vi "MoticApi.vi"() -> ()   [LabVIEW 2012]
uses:
  MoticApi/MoticApi.lvlib
  <vilib>/picture/picture.llb/imagedata.ctl
panel:
  in  "Reset ROI":bool
  in  "Right":i32
  in  "Bottom":i32
  in  "Left":i32
  in  "Top":i32
  out "Max height":i32=486
  out "Max width":i32=648
  out "Bits per component":i32
  out "Components per pixel":i32
  in  "Activate cooler":bool
  out "Cooler available?":bool
  out "Camera connected":bool
  out "Frame format":u32(ring) items=["GRBG", "BGGR", "GBRG", "RGGB", "RGB", "BGR", "Monochrome"]
  out "Camera type":u32(ring) items=["Unknown", "MC1001", "MC2001", "MC3001", "MC2001B", "MC1002", "MC2002", "MA205", "MA285", "MA252", "Swift MC1002", "MD3300: deprecated Since MA252 added", "MC5001", "MC3111", "MC3222", "MC3022", "Swift MC3001", "Swift MC3222", "Swift MC3111", "MA282", "MC352+: Not available at present", "MC3521: Not available at present", "MC10M"]
  in  "Trigger type":u32(ring) items=["Free", "Software", "Hardware-Rise", "Hardware-Fall"]
  out "Temperature data available?":bool
  out "Relative Humidity":dbl
  out "Ambient Temperature":dbl
  out "Sensor temperature":dbl
  in  "Resolution":i32(ring) items=["2592 x 1944", "1296 x 972", "648 x 486"]
  in  "Frequency index":i32(slide)=3 min=0 max=8 step=1 scale=0.0..8.0
  in  "Exposure, ms":sgl(slide)=0.14 min=0.14 max=5674.29 step=1 scale=0.14000000059604645..5674.2919921875
  out "Current height":i32=486
  out "Current width":i32=648
  in  "Acquisition enabled":bool
  in  "Blue Gain":sgl(slide)=1.0 min=1 max=128 step=0.125 scale=1.0..128.0
  in  "Green Gain":sgl(slide)=1.0 min=1 max=128 step=0.125 scale=1.0..128.0
  in  "Red Gain":sgl(slide)=1.0 min=1 max=128 step=0.125 scale=1.0..128.0
  in  "Blue Offset":i32(slide) min=-255 max=255 step=1 scale=-255.0..255.0
  in  "Green Offset":i32(slide) min=-255 max=255 step=1 scale=-255.0..255.0
  in  "Red Offset":i32(slide) min=-255 max=255 step=1 scale=-255.0..255.0
  out "Image":T1(plugin-control)
  in  "stop":bool
  out "2D Picture":picture
  out "height array out":i32[](array[numeric])=[1944, 972, 486]
  out "width array out":i32[](array[numeric])=[2592, 1296, 648]
  out "error out":errorcluster
  # "ROI configuration"
  # "0 - fastest"
  # "Color Gain"
  # "Color Offset"
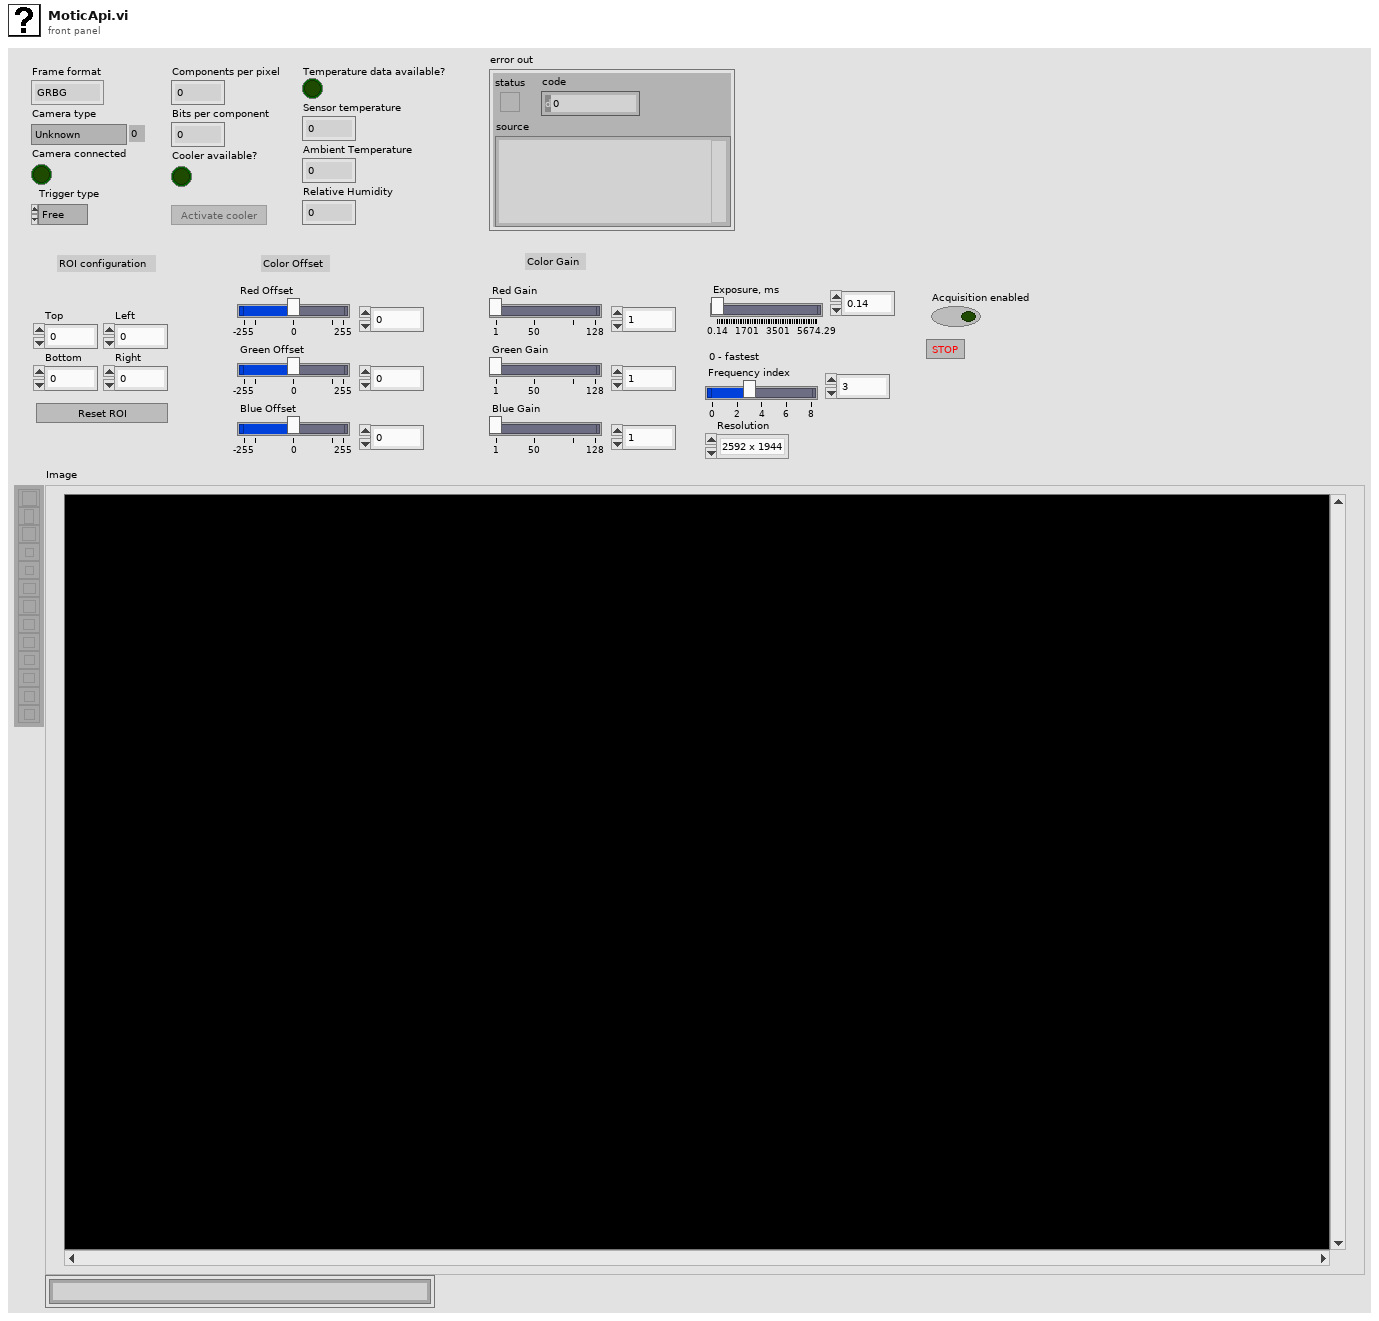
[diagram p1: front panel]
types:
  T1 = typedef "IMAQ Image.ctl" = refnum<image>
  T2 = enum8{"Enabled", "Disabled", "Disabled and Grayed Out"}
  T3 = typedef "Image Type" = u32
  T4 = cluster{"left":i16, "top":i16, "right":i16, "bottom":i16}
  T5 = typedef "imagedata.ctl" = cluster{"image type":i32, "image depth":i32, "image":u8[], "mask":u8[], "colors":u32[], "Rectangle":cluster{"left":i16, "top":i16, "right":i16, "bottom":i16}}
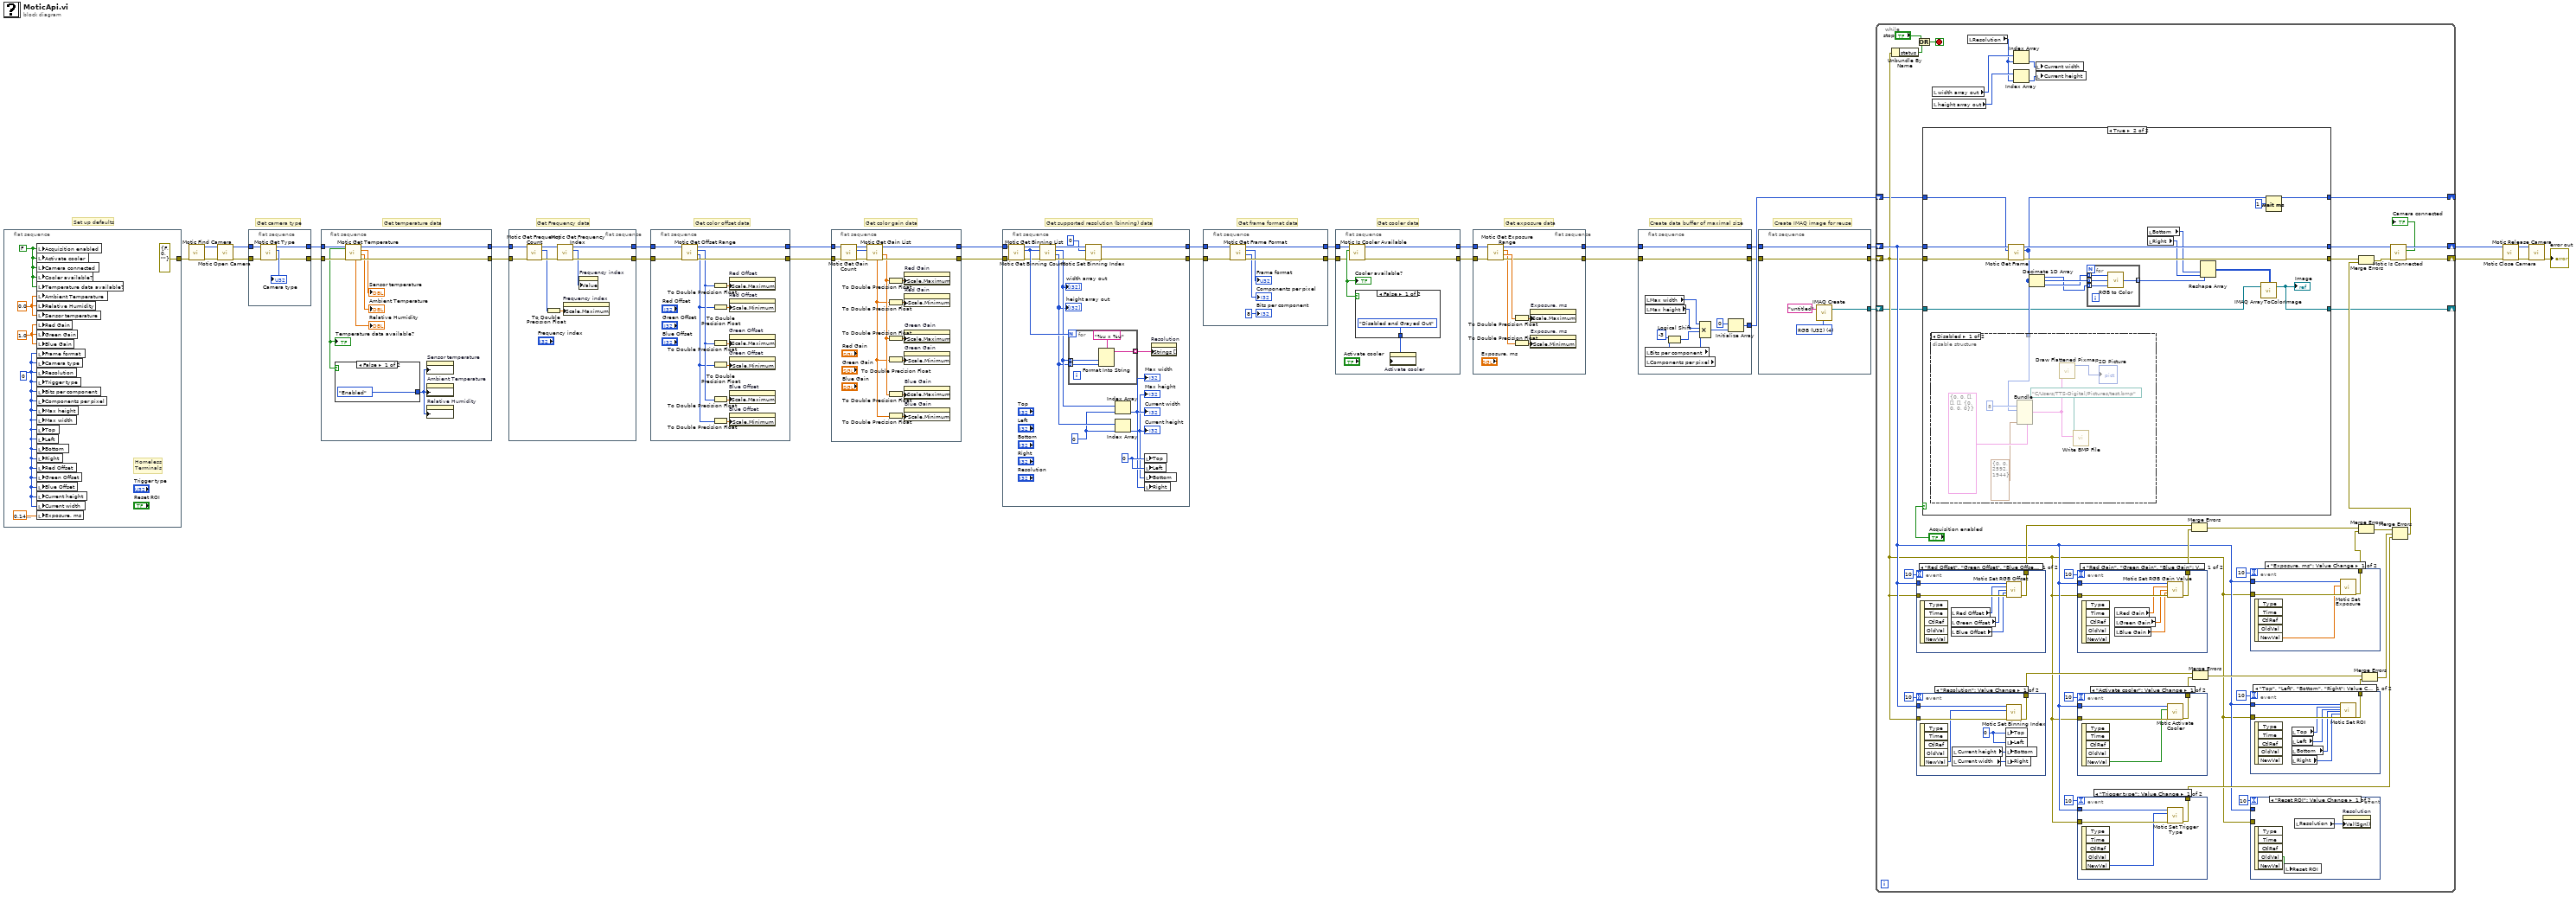
[diagram p0: block diagram]
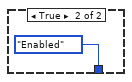
[diagram p2: hidden frame]
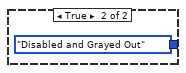
[diagram p3: hidden frame]
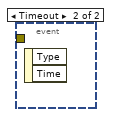
[diagram p4: hidden frame]
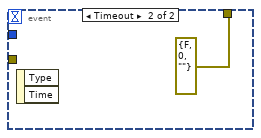
[diagram p5: hidden frame]
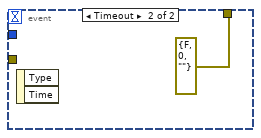
[diagram p6: hidden frame]
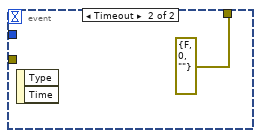
[diagram p7: hidden frame]
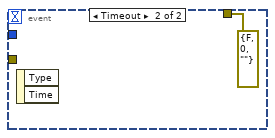
[diagram p8: hidden frame]
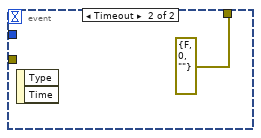
[diagram p9: hidden frame]
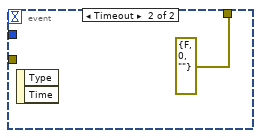
[diagram p10: hidden frame]
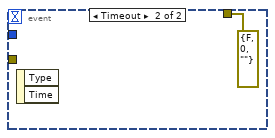
[diagram p13: hidden frame]
diagram:
  # "Set up defaults"
  # "Create IMAQ image for reuse"
  # "Create data buffer of maximal size"
  # "Get camera type"
  # "Get exposure data"
  # "Get cooler data"
  # "Get frame format data"
  # "Get supported resolution (binning) data"
  # "Get color gain data"
  # "Get color offset data"
  # "Get Frequency data"
  # "Get temperature data"
  n1 = flat-sequence {
    tunnel: [errorcluster {"status"=FALSE, "code"=0, "source"=""} ("error in (no error)")] -> w7
    frame #0 {
      w35 = sgl 1.0 ("Red Gain")
      w36 = 0
      w39 = 0.0 ("Ambient Temperature")
      w37 = FALSE ("Acquisition enabled")
      # "Homeless\nTerminals"
      n2 = local write "Acquisition enabled"(w37) -> ()
      n3 = local write "Activate cooler"(w37) -> ()
      n4 = local write "Camera connected"(w37) -> ()
      n5 = local write "Cooler available?"(w37) -> ()
      n6 = local write "Temperature data available?"(w37) -> ()
      n7 = local write "Ambient Temperature"(w39) -> ()
      n8 = local write "Relative Humidity"(w39) -> ()
      n9 = local write "Sensor temperature"(w39) -> ()
      n10 = local write "Red Gain"(w35) -> ()
      n11 = local write "Green Gain"(w35) -> ()
      n12 = local write "Blue Gain"(w35) -> ()
      n13 = local write "Frame format"(w36) -> ()
      n14 = local write "Camera type"(w36) -> ()
      n15 = local write "Resolution"(w36) -> ()
      n16 = local write "Trigger type"(w36) -> ()
      n17 = local write "Bits per component"(w36) -> ()
      n18 = local write "Components per pixel"(w36) -> ()
      n19 = local write "Max height"(w36) -> ()
      n20 = local write "Max width"(w36) -> ()
      n21 = local write "Top"(w36) -> ()
      n22 = local write "Left"(w36) -> ()
      n23 = local write "Bottom"(w36) -> ()
      n24 = local write "Right"(w36) -> ()
      n25 = local write "Red Offset"(w36) -> ()
      n26 = local write "Green Offset"(w36) -> ()
      n27 = local write "Blue Offset"(w36) -> ()
      n28 = local write "Current height"(w36) -> ()
      n29 = local write "Current width"(w36) -> ()
      n30 = local write "Exposure, ms"(sgl 0.14 ("Exposure, ms")) -> ()
    }
  }
  n31 = call "Motic Find Camera.vi"("error in (no error)"=w7) -> ("error out"=w14:errorcluster, "camera out"=w17:i32)  [unwired: 9 in]
  n32 = call "Motic Open Camera.vi"("error in (no error)"=w14, "camera"=w17) -> ("error out"=w15:errorcluster, "camera out"=w16:i32)  [unwired: 8 in]
  n33 = flat-sequence {
    tunnel: [w44] -> w19
    tunnel: [w43] -> w18
    tunnel: w16 -> [w42]
    tunnel: w15 -> [w41]
    frame #0 {
      n34 = call "Motic Get Type.vi"("error in (no error)"=w41, "camera"=w42) -> ("error out"=w43:errorcluster, "camera type"=→"Camera type":u32, "camera out"=w44:i32)  [unwired: 7 in]
    }
  }
  n35 = flat-sequence {
    tunnel: w19 -> [w54]
    tunnel: w18 -> [w53]
    tunnel: [w52] -> w25
    tunnel: [w51] -> w24
    frame #0 {
      n36 = call "Motic Get Temperature.vi"("error in (no error)"=w53, "camera"=w54) -> ("error out"=w51:errorcluster, "ambient temperature out"=→"Ambient Temperature":sgl, "sensor surface temperature out"=→"Sensor temperature":sgl, "camera out"=w52:i32, "relative humidity out"=→"Relative Humidity":sgl, "is temperature data available?"=w47:bool)  [unwired: 4 in]
      "Temperature data available?" <- w47
      n37 = case shown="False" w47 {
        tunnel: [T2."Enabled" ("Disabled") T2."Disabled and Grayed Out" ("Disabled")] -> w46
        frame False {
        }
        frame True {
        }
      }
      n38 = property on="Sensor temperature" class="DigNum (strict)"("DisabledEnum"=w46) -> ()  [unwired: 2 in, 2 out]
      n39 = property on="Ambient Temperature" class="DigNum (strict)"("DisabledEnum"=w46) -> ()  [unwired: 2 in, 2 out]
      n40 = property on="Relative Humidity" class="DigNum (strict)"("DisabledEnum"=w46) -> ()  [unwired: 2 in, 2 out]
    }
  }
  n41 = flat-sequence {
    tunnel: [w63] -> w27
    tunnel: [w62] -> w26
    tunnel: w25 -> [w58]
    tunnel: w24 -> [w57]
    frame #0 {
      n42 = call "Motic Get Frequency Count.vi"("error in (no error)"=w57, "camera"=w58) -> ("error out"=w64:errorcluster, "frequency count"=w60:i32, "camera out"=w65:i32)  [unwired: 7 in]
      n43 = To Double Precision Float(number=w60) -> (double precision float=w61:dbl)
      n44 = call "Motic Get Frequency Index.vi"("error in (no error)"=w64, "camera"=w65) -> ("error out"=w62:errorcluster, "frequency index"=w59:i32, "camera out"=w63:i32)  [unwired: 7 in]
      n45 = property on="Frequency index" class="Slide (strict)"("Scale.Maximum"=w61) -> ()  [unwired: 2 in, 2 out]
      n46 = property on="Frequency index" class="Slide (strict)"("Value"=w59) -> ()  [unwired: 2 in, 2 out]
    }
  }
  n47 = flat-sequence {
    tunnel: [w77] -> w2
    tunnel: [w76] -> w1
    tunnel: w27 -> [w67]
    tunnel: w26 -> [w66]
    frame #0 {
      n48 = call "Motic Get Offset Range.vi"("error in (no error)"=w66, "camera"=w67) -> ("error out"=w76:errorcluster, "min out"=w68:i32, "max out"=w69:i32, "camera out"=w77:i32)  [unwired: 6 in]
      n49 = To Double Precision Float(number=w69) -> (double precision float=w74:dbl)
      n50 = To Double Precision Float(number=w68) -> (double precision float=w75:dbl)
      n51 = To Double Precision Float(number=w69) -> (double precision float=w72:dbl)
      n52 = To Double Precision Float(number=w68) -> (double precision float=w73:dbl)
      n53 = To Double Precision Float(number=w69) -> (double precision float=w70:dbl)
      n54 = To Double Precision Float(number=w68) -> (double precision float=w71:dbl)
      n55 = property on="Red Offset" class="Slide (strict)"("Scale.Maximum"=w74) -> ()  [unwired: 2 in, 2 out]
      n56 = property on="Red Offset" class="Slide (strict)"("Scale.Minimum"=w75) -> ()  [unwired: 2 in, 2 out]
      n57 = property on="Green Offset" class="Slide (strict)"("Scale.Maximum"=w72) -> ()  [unwired: 2 in, 2 out]
      n58 = property on="Green Offset" class="Slide (strict)"("Scale.Minimum"=w73) -> ()  [unwired: 2 in, 2 out]
      n59 = property on="Blue Offset" class="Slide (strict)"("Scale.Maximum"=w70) -> ()  [unwired: 2 in, 2 out]
      n60 = property on="Blue Offset" class="Slide (strict)"("Scale.Minimum"=w71) -> ()  [unwired: 2 in, 2 out]
    }
  }
  n61 = flat-sequence {
    tunnel: w2 -> [w92]
    tunnel: w1 -> [w91]
    tunnel: [w81] -> w3
    tunnel: [w80] -> w4
    frame #0 {
      n62 = call "Motic Get Gain Count.vi"("error in (no error)"=w91, "camera"=w92) -> ("error out"=w88:errorcluster, "gain count"=w90:i32, "camera out"=w89:i32)  [unwired: 7 in]
      n63 = call "Motic Get Gain List.vi"("error in (no error)"=w88, "gain count"=w90, "camera"=w89) -> ("error out"=w81:errorcluster, "max gain"=w79:sgl, "camera out"=w80:i32, "min gain"=w78:sgl)  [unwired: 4 in, 1 out]
      n64 = To Double Precision Float(number=w79) -> (double precision float=w86:dbl)
      n65 = To Double Precision Float(number=w78) -> (double precision float=w87:dbl)
      n66 = To Double Precision Float(number=w79) -> (double precision float=w84:dbl)
      n67 = To Double Precision Float(number=w78) -> (double precision float=w85:dbl)
      n68 = To Double Precision Float(number=w79) -> (double precision float=w82:dbl)
      n69 = To Double Precision Float(number=w78) -> (double precision float=w83:dbl)
      n70 = property on="Red Gain" class="Slide (strict)"("Scale.Maximum"=w86) -> ()  [unwired: 2 in, 2 out]
      n71 = property on="Red Gain" class="Slide (strict)"("Scale.Minimum"=w87) -> ()  [unwired: 2 in, 2 out]
      n72 = property on="Green Gain" class="Slide (strict)"("Scale.Maximum"=w84) -> ()  [unwired: 2 in, 2 out]
      n73 = property on="Green Gain" class="Slide (strict)"("Scale.Minimum"=w85) -> ()  [unwired: 2 in, 2 out]
      n74 = property on="Blue Gain" class="Slide (strict)"("Scale.Maximum"=w82) -> ()  [unwired: 2 in, 2 out]
      n75 = property on="Blue Gain" class="Slide (strict)"("Scale.Minimum"=w83) -> ()  [unwired: 2 in, 2 out]
    }
  }
  n76 = flat-sequence {
    tunnel: [w105] -> w23
    tunnel: [w104] -> w22
    tunnel: w4 -> [w101]
    tunnel: w3 -> [w100]
    frame #0 {
      w95 = 0 ("index")
      w96 = 0 ("Top")
      n77 = call "Motic Get Binning Count.vi"("error in (no error)"=w100, "camera"=w101) -> ("error out"=w102:errorcluster, "binning count"=w106:i32, "camera out"=w103:i32)  [unwired: 7 in]
      n78 = call "Motic Get Binning List.vi"("error in (no error)"=w102, "binning count"=w106, "camera"=w103) -> ("error out"=w108:errorcluster, "height array out"=w97:i32[], "width array out"=w98:i32[], "camera out"=w109:i32)  [unwired: 5 in]
      "width array out" <- w98
      "height array out" <- w97
      n79 = for {
        N: w106 -> [_]
        tunnel: w98 -> [w112] mode=indexing
        tunnel: w97 -> [w111] mode=indexing
        tunnel: [w110] -> w99 mode=indexing
        n80 = Format Into String(format string="%u x %u", w112, w111) -> (resulting string=w110:string)  [unwired: 2 in, 1 out]
      }
      n81 = call "Motic Set Binning Index.vi"("error in (no error)"=w108, "idx"=0, "camera"=w109) -> ("error out"=w104:errorcluster, "camera out"=w105:i32)  [unwired: 7 in]
      n82 = Index Array(array=w98, index=w95) -> (element=w94:i32)
      "Current width" <- w94
      "Max width" <- w94
      n83 = Index Array(array=w97, index=w95) -> (element=w93:i32)
      "Current height" <- w93
      "Max height" <- w93
      n84 = local write "Top"(w96) -> ()
      n85 = local write "Left"(w96) -> ()
      n86 = local write "Bottom"(w93) -> ()
      n87 = local write "Right"(w94) -> ()
      n88 = property on="Resolution" class="Ring (strict)"("Strings []"=w99) -> ()  [unwired: 2 in, 2 out]
    }
  }
  n89 = flat-sequence {
    tunnel: w23 -> [w120]
    tunnel: w22 -> [w119]
    tunnel: [w118] -> w21
    tunnel: [w117] -> w20
    frame #0 {
      n90 = call "Motic Get Frame Format.vi"("error in (no error)"=w119, "camera"=w120) -> ("error out"=w117:errorcluster, "components per pixel"=→"Components per pixel":i32, "frame format"=→"Frame format":u32, "camera out"=w118:i32)  [unwired: 6 in]
      "Bits per component" <- 8 ("bits per component")
    }
  }
  n91 = flat-sequence {
    tunnel: [w126] -> w29
    tunnel: [w125] -> w28
    tunnel: w21 -> [w123]
    tunnel: w20 -> [w122]
    frame #0 {
      n92 = call "Motic Is Cooler Available.vi"("error in (no error)"=w122, "camera"=w123) -> ("error out"=w125:errorcluster, "cooler available?"=w124:bool, "camera out"=w126:i32)  [unwired: 7 in]
      "Cooler available?" <- w124
      n93 = case shown="False" w124 {
        tunnel: [T2."Disabled and Grayed Out" ("Disabled") T2."Enabled" ("Disabled")] -> w121
        frame False {
        }
        frame True {
        }
      }
      n94 = property on="Activate cooler" class="Bool (strict)"("DisabledEnum"=w121) -> ()  [unwired: 2 in, 2 out]
    }
  }
  n95 = flat-sequence {
    tunnel: [w133] -> w6
    tunnel: [w132] -> w5
    tunnel: w29 -> [w130]
    tunnel: w28 -> [w129]
    frame #0 {
      n96 = call "Motic Get Exposure Range.vi"("error in (no error)"=w129, "camera"=w130) -> ("error out"=w132:errorcluster, "range max"=w134:sgl, "range min"=w131:sgl, "camera out"=w133:i32)  [unwired: 6 in]
      n97 = To Double Precision Float(number=w134) -> (double precision float=w135:dbl)
      n98 = To Double Precision Float(number=w131) -> (double precision float=w136:dbl)
      n99 = property on="Exposure, ms" class="Slide (strict)"("Scale.Maximum"=w135) -> ()  [unwired: 2 in, 2 out]
      n100 = property on="Exposure, ms" class="Slide (strict)"("Scale.Minimum"=w136) -> ()  [unwired: 2 in, 2 out]
    }
  }
  n101 = flat-sequence {
    tunnel: [w147] -> w12
    tunnel: [w146] -> w11
    tunnel: w6 -> [w147]
    tunnel: w5 -> [w146]
    tunnel: [w137] -> w13
    frame #0 {
      n102 = local read "Max width"() -> (w141:i32)
      n103 = local read "Max height"() -> (w138:i32)
      n104 = local read "Bits per component"() -> (w139:i32)
      n105 = local read "Components per pixel"() -> (w140:i32)
      n106 = Logical Shift(y=-3, x=w139) -> (x << y=w143:i32)
      n107 = Compound Arithmetic op=MULTIPLY(w141, w138, w143, w140) -> (w144:i32)
      n108 = Initialize Array(u8 0 ("element"), w144) -> (w137:u8[])
    }
  }
  n109 = flat-sequence {
    tunnel: [w152] -> w10
    tunnel: [w151] -> w9
    tunnel: w12 -> [w152]
    tunnel: w11 -> [w151]
    tunnel: [w148] -> w8
    frame #0 {
      w150 = T3 4 items=["Grayscale (U8)", "Grayscale (I16)", "Grayscale (SGL)", "Complex (CSG)", "RGB (U32)", "HSL (U32)", "RGB (U64)", "Grayscale (U16)"] ("Image Type")
      n110 = call "IMAQ Create"("Image Name"="untitled", "Image Type"=w150) -> ("New Image"=w148:T1)  [unwired: 3 in, 1 out]
    }
  }
  n111 = while {
    shift-right: [w178] -> w31
    shift-left: w10 -> [w167]
    shift-right: [w180] -> w30
    shift-left: w9 -> [w160]
    shift-right: [w155] -> _
    shift-left: w13 -> [w156]
    shift-right: [w153] -> _
    shift-left: w8 -> [w154]
    stop <- w157 stop-if-true
    n112 = Unbundle By Name(w160) -> ("status"=w159:bool)
    n113 = Or(x="stop", y=w159) -> (x .or. y?=w157:bool)
    n114 = event shown="[0] \"Red Offset\", \"Green Offset\", \"Blue Offset\": Value Change" {
      selector: _ -> [_ _]
      dyn-events: _ -> [_ _]
      timeout: 10 -> [_ _]
      tunnel: w167 -> [w270 _]
      tunnel: w160 -> [w269 _]
      tunnel: [w268 errorcluster {"status"=FALSE, "code"=0, "source"=""} ("error out")] -> w188
      event "Red Offset", "Green Offset", "Blue Offset": Value Change {
        n115 = event-data() -> ()  [unwired: 1 in, 5 out]
        n116 = local read "Red Offset"() -> (w267:i32)
        n117 = local read "Green Offset"() -> (w266:i32)
        n118 = local read "Blue Offset"() -> (w265:i32)
        n119 = call "Motic Set RGB Offset.vi"("camera"=w270, "r"=w267, "g"=w266, "b"=w265, "error in (no error)"=w269) -> ("error out"=w268:errorcluster)  [unwired: 9 in, 1 out]
      }
      event Timeout {
        n120 = event-data() -> ()  [unwired: 1 in, 2 out]
      }
    }
    n121 = event shown="[0] \"Resolution\": Value Change" {
      selector: _ -> [_ _]
      dyn-events: _ -> [_ _]
      timeout: 10 -> [_ _]
      tunnel: w167 -> [w220 _]
      tunnel: w160 -> [w219 _]
      tunnel: [w218 errorcluster {"status"=FALSE, "code"=0, "source"=""} ("error out")] -> w175
      event "Resolution": Value Change {
        w216 = 0 ("Top")
        n122 = event-data() -> ("NewVal"=w217:i32)  [unwired: 1 in, 4 out]
        n123 = local read "Current height"() -> (w215:i32)
        n124 = local read "Current width"() -> (w214:i32)
        n125 = local write "Top"(w216) -> ()
        n126 = local write "Left"(w216) -> ()
        n127 = local write "Bottom"(w215) -> ()
        n128 = local write "Right"(w214) -> ()
        n129 = call "Motic Set Binning Index.vi"("error in (no error)"=w219, "idx"=w217, "camera"=w220) -> ("error out"=w218:errorcluster)  [unwired: 7 in, 1 out]
      }
      event Timeout {
        n130 = event-data() -> ()  [unwired: 1 in, 2 out]
      }
    }
    n131 = case shown="True" "Acquisition enabled" {
      tunnel: [w237 w253] -> w179
      tunnel: [w236 w252] -> w191
      tunnel: w167 -> [w237 w251]
      tunnel: w160 -> [w236 w250]
      tunnel: w156 -> [w235 w241]
      tunnel: [w235 w240] -> w155
      tunnel: w154 -> [w234 w239]
      tunnel: [w234 w238] -> w153
      frame False {
      }
      frame True {
        n132 = call "Motic Get Frame.vi"("error in (no error)"=w250, "image buffer in"=w241, "camera"=w251) -> ("error out"=w252:errorcluster, "image buffer out"=w240:u8[], "camera out"=w253:i32)  [unwired: 5 in, 1 out]
        n133 = disable-structure shown="Disabled" {
          disable-tunnel: w240 -> [w254 _]
          frame Disabled {
            n134 = Bundle(cluster=T5 {"image type"=0, "image depth"=0, "image"=[], "mask"=[], "colors"=[], "Rectangle"={"left"=0, "top"=0, "right"=0, "bottom"=0}} ("image data"), "image depth"=8, "image"=w254, "Rectangle"=T4 {"left"=0, "top"=0, "right"=2592, "bottom"=1944}) -> (w258:T5)  [unwired: 3 in]
            n135 = call <vilib>:"Draw Flattened Pixmap.vi"("image data"=w258) -> ("new picture"=→"2D Picture":picture)  [unwired: 8 in]
            n136 = call <vilib>:"Write BMP File.vi"("image data"=w258, "path to BMP file"=path "C:/Users/TTS-Digital/Pictures/test.bmp") -> ()  [unwired: 8 in, 2 out]
          }
          frame Enabled {
          }
        }
        n137 = Decimate 1D Array(w240) -> (w247:u8[], w249:u8[], w248:u8[])
        n138 = for {
          tunnel: w249 -> [w263] mode=indexing
          tunnel: w247 -> [w264] mode=indexing
          tunnel: w248 -> [w262] mode=indexing
          tunnel: [w261] -> w246 mode=indexing
          n139 = call <vilib>:"RGB to Color.vi"("B"=w264, "G"=w263, "R"=w262) -> ("Color"=w261:u32)
        }
        n140 = local read "Bottom"() -> (w243:i32)
        n141 = local read "Right"() -> (w242:i32)
        n142 = Reshape Array(w246, w243, w242) -> (w245:u32[][])
        n143 = call "IMAQ ArrayToColorImage"("Image Pixels (U32)"=w245, "Image"=w239) -> ("Image Out"=w238:T1)  [unwired: 3 in, 1 out]
        "Image" <- w238
        n144 = Wait (ms)(milliseconds to wait=u32 1) -> ()  [unwired: 1 out]
      }
    }
    n145 = local read "width array out"() -> (w165:i32[])
    n146 = local read "height array out"() -> (w164:i32[])
    n147 = local read "Resolution"() -> (w163:i32)
    n148 = Index Array(array=w165, index=w163) -> (element=w162:i32)
    n149 = Index Array(array=w164, index=w163) -> (element=w161:i32)
    n150 = local write "Current width"(w162) -> ()
    n151 = local write "Current height"(w161) -> ()
    n152 = event shown="[0] \"Red Gain\", \"Green Gain\", \"Blue Gain\": Value Change" {
      selector: _ -> [_ _]
      dyn-events: _ -> [_ _]
      timeout: 10 -> [_ _]
      tunnel: w167 -> [w232 _]
      tunnel: w160 -> [w231 _]
      tunnel: [w230 errorcluster {"status"=FALSE, "code"=0, "source"=""} ("error out")] -> w189
      event "Red Gain", "Green Gain", "Blue Gain": Value Change {
        n153 = event-data() -> ()  [unwired: 1 in, 5 out]
        n154 = local read "Red Gain"() -> (w229:sgl)
        n155 = local read "Green Gain"() -> (w228:sgl)
        n156 = local read "Blue Gain"() -> (w227:sgl)
        n157 = call "Motic Set RGB Gain Value.vi"("camera"=w232, "r"=w229, "g"=w228, "b"=w227, "error in (no error)"=w231) -> ("error out"=w230:errorcluster)  [unwired: 6 in, 4 out]
      }
      event Timeout {
        n158 = event-data() -> ()  [unwired: 1 in, 2 out]
      }
    }
    n159 = event shown="[0] \"Activate cooler\": Value Change" {
      selector: _ -> [_ _]
      dyn-events: _ -> [_ _]
      timeout: 10 -> [_ _]
      tunnel: w167 -> [w212 _]
      tunnel: w160 -> [w211 _]
      tunnel: [w210 errorcluster {"status"=FALSE, "code"=0, "source"=""} ("error out")] -> w176
      event "Activate cooler": Value Change {
        n160 = event-data() -> ("NewVal"=w209:bool)  [unwired: 1 in, 4 out]
        n161 = call "Motic Activate Cooler.vi"("error in (no error)"=w211, "activate"=w209, "camera"=w212) -> ("error out"=w210:errorcluster)  [unwired: 6 in, 2 out]
      }
      event Timeout {
        n162 = event-data() -> ()  [unwired: 1 in, 2 out]
      }
    }
    n163 = event shown="[0] \"Trigger type\": Value Change" {
      selector: _ -> [_ _]
      dyn-events: _ -> [_ _]
      timeout: 10 -> [_ _]
      tunnel: w167 -> [w199 _]
      tunnel: w160 -> [w198 _]
      tunnel: [w197 errorcluster {"status"=FALSE, "code"=0, "source"=""} ("error out")] -> w168
      event "Trigger type": Value Change {
        n164 = event-data() -> ("NewVal"=w196:u32)  [unwired: 1 in, 4 out]
        n165 = call "Motic Set Trigger Type.vi"("error in (no error)"=w198, "trigger type"=w196, "camera"=w199) -> ("error out"=w197:errorcluster)  [unwired: 7 in, 1 out]
      }
      event Timeout {
        n166 = event-data() -> ()  [unwired: 1 in, 2 out]
      }
    }
    n167 = Merge Errors(w188, w189) -> (w186:errorcluster)
    n168 = Merge Errors(w175, w176) -> (w174:errorcluster)
    n169 = event shown="[0] \"Exposure, ms\": Value Change" {
      selector: _ -> [_ _]
      dyn-events: _ -> [_ _]
      timeout: 10 -> [_ _]
      tunnel: w167 -> [w225 _]
      tunnel: w160 -> [w224 _]
      tunnel: [w223 errorcluster {"status"=FALSE, "code"=0, "source"=""} ("error out")] -> w185
      event "Exposure, ms": Value Change {
        n170 = event-data() -> ("NewVal"=w222:sgl)  [unwired: 1 in, 4 out]
        n171 = call "Motic Set Exposure.vi"("error in (no error)"=w224, "exposure"=w222, "camera"=w225) -> ("error out"=w223:errorcluster)  [unwired: 7 in, 1 out]
      }
      event Timeout {
        n172 = event-data() -> ()  [unwired: 1 in, 2 out]
      }
    }
    n173 = event shown="[0] \"Top\", \"Left\", \"Bottom\", \"Right\": Value Change" {
      selector: _ -> [_ _]
      dyn-events: _ -> [_ _]
      timeout: 10 -> [_ _]
      tunnel: w167 -> [w207 _]
      tunnel: w160 -> [w206 _]
      tunnel: [w205 errorcluster {"status"=FALSE, "code"=0, "source"=""} ("error out")] -> w173
      event "Top", "Left", "Bottom", "Right": Value Change {
        n174 = event-data() -> ()  [unwired: 1 in, 5 out]
        n175 = local read "Top"() -> (w204:i32)
        n176 = local read "Left"() -> (w203:i32)
        n177 = local read "Bottom"() -> (w202:i32)
        n178 = local read "Right"() -> (w201:i32)
        n179 = call "Motic Set ROI.vi"("camera"=w207, "top"=w204, "left"=w203, "bottom"=w202, "right"=w201, "error in (no error)"=w206) -> ("error out"=w205:errorcluster)  [unwired: 8 in, 5 out]
      }
      event Timeout {
        n180 = event-data() -> ()  [unwired: 1 in, 2 out]
      }
    }
    n181 = event shown="[0] \"Reset ROI\": Value Change" {
      selector: _ -> [_ _]
      dyn-events: _ -> [_ _]
      timeout: 10 -> [_ _]
      tunnel: w167 -> [_ _]
      tunnel: w160 -> [_ _]
      event "Reset ROI": Value Change {
        n182 = event-data() -> ("OldVal"=w195:bool)  [unwired: 1 in, 4 out]
        n183 = local write "Reset ROI"(w195) -> ()
        n184 = local read "Resolution"() -> (w194:i32)
        n185 = property on="Resolution" class="Ring (strict)"("Val(Sgnl)"=w194) -> ()  [unwired: 2 in, 2 out]
      }
      event Timeout {
        n186 = event-data() -> ()  [unwired: 1 in, 2 out]
      }
    }
    n187 = Merge Errors(w186, w185) -> (w171:errorcluster)
    n188 = Merge Errors(w174, w173) -> (w172:errorcluster)
    n189 = Merge Errors(w171, w172, w168) -> (w170:errorcluster)
    n190 = Merge Errors(w191, w170) -> (w181:errorcluster)
    n191 = call "Motic Is Connected.vi"("error in (no error)"=w181, "camera"=w179) -> ("error out"=w180:errorcluster, "is connected?"=→"Camera connected":bool, "camera out"=w178:i32)  [unwired: 7 in]
  }
  n192 = call "Motic Close Camera.vi"("error in (no error)"=w30, "camera"=w31) -> ("error out"=w32:errorcluster, "camera out"=w33:i32)  [unwired: 8 in]
  n193 = call "Motic Release Camera.vi"("error in (no error)"=w32, "camera"=w33) -> ("error out"=→"error out":errorcluster)  [unwired: 9 in]
